vi "Winkel_ISO_bestimmen.vi"(8 "Fehler in":errorcluster, 11 "Cluster in":T1={"Initialisierung"={"Online?"=FALSE, "Grundpfad"=path "", "Kamera Oben"="", "IP-Adresse Flüssiglinse"="", "Flüssiglinse"=refnum, "Kamera Unten"="", "IP-Adresse SPS"="", "SPS-Verbindung"={"TCP Connection Ref"=refnum, "IP address"="", "timeout ms"=5000, "Connected?"=FALSE, "PLC Type"=enum."S7 1200", "Rack S7 400"=0, "Slot S7 400"=0, "PDU Size"=0, "connection semaphore"=refnum}, "IP-Adresse Lichtgitter"="", "Lichtgitter"=refnum, "Skalierungsfaktor"=0.0, "Bilder Oben"=[], "Bild Unten"=refnum, "Bild Ausschnitt Unten"=refnum}, "Einstellungen"={"Gesamtablauf gestartet"=FALSE, "i. O. Bilder speichern"=FALSE, "Bildspeicherung Offline"=FALSE, "Ausgewähltes Offline-Datum"="", "Ausgewähltes Offline-Teil"="", "Speicherpfad Bilder"=path ""}, "Artikeldaten"={"Artikelnummer"="", "Fertigungsauftrag"="", "Muster ISO"=refnum, "Belichtungszeit Referenzmarken"=0.0, "Fokus Referenzmarken"=0.0, "Belichtungszeit ISO"=0.0, "Fokus ISO"=0.0, "Belichtungszeit Unten"=0.0, "Kontaktanzahl"=0, "Aktueller Kontakt"=0, "Kontaktposition"={"x"=0.0, "y"=0.0}, "ISO-Muster nicht vorhanden"=FALSE, "Winkel ISO"=0.0, "Mittelpunkt ISO"={"x"=0.0, "y"=0.0}}, "Werte Kamera Oben"={"Koordinatensystem"={"Punkt x-Achse"={"X"=0.0, "Y"=0.0}, "Ursprung"={"X"=0.0, "Y"=0.0}, "Punkt y-Achse"={"X"=0.0, "Y"=0.0}}, "Position Kontakt"={"x"=0.0, "y"=0.0}, "Durchmesser Loch"=0.0, "Winkel Kontakt"=0.0, "Position Kontakt umgerechnet"={"x"=0.0, "y"=0.0}}, "Werte Kamera Unten"={"Prüfung Unten n. i. O."=FALSE}, "Werte Lichtgitter"={"Messwerte Referenzmarken"=[], "Mittelpunkt Referenzmarken"={"x"=0.0, "y"=0.0}, "Messwerte Kontakt"=[], "Offset"={"x"=0.0, "y"=0.0}}, "Rückmeldungen"={"Koordinaten ermittelt"=FALSE, "Vermessung Lichtgitter fertig"=FALSE, "Nachkontrolle Kamera Unten fertig"=FALSE}, "Fehler"={"Referenzen nicht gefunden"=FALSE, "Kontakt nicht gefunden"=FALSE, "Referenzen nicht in Lichtgitter"=FALSE, "Kontakt zu groß"=FALSE, "Kontakt zu klein"=FALSE}, "Statistik"={"Statistiken"=[]}, "Timer"={"Timer Start Position"=0, "Timer Start Lichtgitter"=0, "Timer Start Kamera Unten"=0}}) -> (0 "Fehler out":errorcluster, 2 "Polbild i.O.":bool, 3 "Cluster out":T1={"Initialisierung"={"Online?"=FALSE, "Grundpfad"=path "", "Kamera Oben"="", "IP-Adresse Flüssiglinse"="", "Flüssiglinse"=refnum, "Kamera Unten"="", "IP-Adresse SPS"="", "SPS-Verbindung"={"TCP Connection Ref"=refnum, "IP address"="", "timeout ms"=5000, "Connected?"=FALSE, "PLC Type"=enum."S7 1200", "Rack S7 400"=0, "Slot S7 400"=0, "PDU Size"=0, "connection semaphore"=refnum}, "IP-Adresse Lichtgitter"="", "Lichtgitter"=refnum, "Skalierungsfaktor"=0.0, "Bilder Oben"=[], "Bild Unten"=refnum, "Bild Ausschnitt Unten"=refnum}, "Einstellungen"={"Gesamtablauf gestartet"=FALSE, "i. O. Bilder speichern"=FALSE, "Bildspeicherung Offline"=FALSE, "Ausgewähltes Offline-Datum"="", "Ausgewähltes Offline-Teil"="", "Speicherpfad Bilder"=path ""}, "Artikeldaten"={"Artikelnummer"="", "Fertigungsauftrag"="", "Muster ISO"=refnum, "Belichtungszeit Referenzmarken"=0.0, "Fokus Referenzmarken"=0.0, "Belichtungszeit ISO"=0.0, "Fokus ISO"=0.0, "Belichtungszeit Unten"=0.0, "Kontaktanzahl"=0, "Aktueller Kontakt"=0, "Kontaktposition"={"x"=0.0, "y"=0.0}, "ISO-Muster nicht vorhanden"=FALSE, "Winkel ISO"=0.0, "Mittelpunkt ISO"={"x"=0.0, "y"=0.0}}, "Werte Kamera Oben"={"Koordinatensystem"={"Punkt x-Achse"={"X"=0.0, "Y"=0.0}, "Ursprung"={"X"=0.0, "Y"=0.0}, "Punkt y-Achse"={"X"=0.0, "Y"=0.0}}, "Position Kontakt"={"x"=0.0, "y"=0.0}, "Durchmesser Loch"=0.0, "Winkel Kontakt"=0.0, "Position Kontakt umgerechnet"={"x"=0.0, "y"=0.0}}, "Werte Kamera Unten"={"Prüfung Unten n. i. O."=FALSE}, "Werte Lichtgitter"={"Messwerte Referenzmarken"=[], "Mittelpunkt Referenzmarken"={"x"=0.0, "y"=0.0}, "Messwerte Kontakt"=[], "Offset"={"x"=0.0, "y"=0.0}}, "Rückmeldungen"={"Koordinaten ermittelt"=FALSE, "Vermessung Lichtgitter fertig"=FALSE, "Nachkontrolle Kamera Unten fertig"=FALSE}, "Fehler"={"Referenzen nicht gefunden"=FALSE, "Kontakt nicht gefunden"=FALSE, "Referenzen nicht in Lichtgitter"=FALSE, "Kontakt zu groß"=FALSE, "Kontakt zu klein"=FALSE}, "Statistik"={"Statistiken"=[]}, "Timer"={"Timer Start Position"=0, "Timer Start Lichtgitter"=0, "Timer Start Kamera Unten"=0}})   [LabVIEW 2024]
uses:
  Typdefinitionen/Cluster.ctl
  <vilib>/userDefined/High Color/IMAQdx.ctl
  <vilib>/DATA AHEAD/SP7/typedefs/S7 Connection.ctl
  <vilib>/DATA AHEAD/SP7/typedefs/PLC Type.ctl
  <vilib>/vision/Image Controls.llb/IMAQ Image.ctl
  Typdefinitionen/Koordinatensystem.ctl
  Typdefinitionen/Statistik.ctl
  <vilib>/vision/NI_Vision_Development_Module.lvlib
  <vilib>/DATA AHEAD/SP7/SP7.lvlib
panel:
  out "Number of Matches":i32
  out "Zeit Pattern Matching":u32
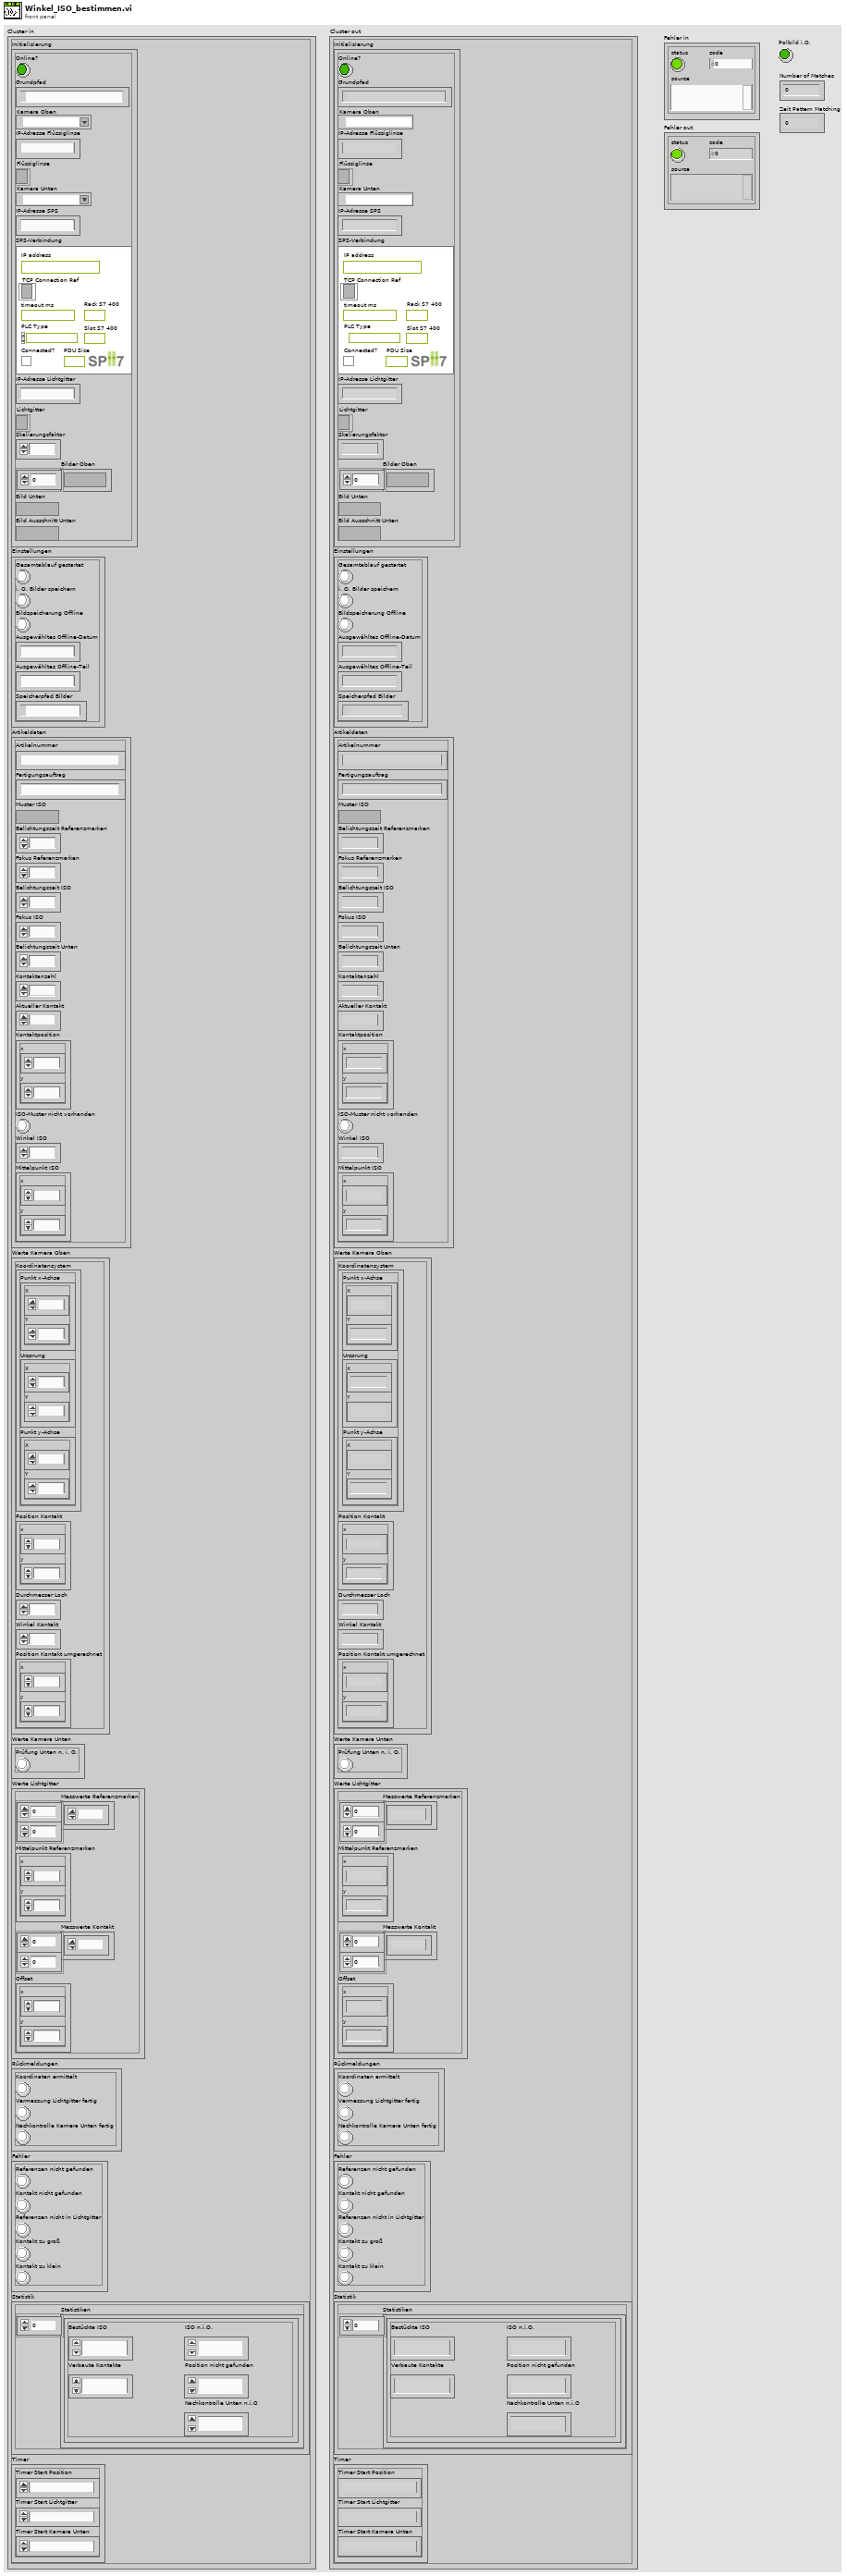
[diagram p1: front panel]
types:
  T1 = typedef "Cluster.ctl" = cluster{"Initialisierung":cluster{"Online?":bool, "Grundpfad":path, "Kamera Oben":T2, "IP-Adresse Flüssiglinse":string, "Flüssiglinse":refnum<k5>, "Kamera Unten":T2, "IP-Adresse SPS":string, "SPS-Verbindung":T3, "IP-Adresse Lichtgitter":string, "Lichtgitter":refnum<k5>, "Skalierungsfaktor":dbl, "Bilder Oben":T6[], "Bild Unten":T6, "Bild Ausschnitt Unten":T6}, "Einstellungen":cluster{"Gesamtablauf gestartet":bool, "i. O. Bilder speichern":bool, "Bildspeicherung Offline":bool, "Ausgewähltes Offline-Datum":string, "Ausgewähltes Offline-Teil":string, "Speicherpfad Bilder":path}, "Artikeldaten":cluster{"Artikelnummer":string, "Fertigungsauftrag":string, "Muster ISO":T6, "Belichtungszeit Referenzmarken":dbl, "Fokus Referenzmarken":dbl, "Belichtungszeit ISO":dbl, "Fokus ISO":dbl, "Belichtungszeit Unten":dbl, "Kontaktanzahl":u32, "Aktueller Kontakt":i16, "Kontaktposition":cluster{"x":sgl, "y":sgl}, "ISO-Muster nicht vorhanden":bool, "Winkel ISO":sgl, "Mittelpunkt ISO":cluster{"x":dbl, "y":dbl}}, "Werte Kamera Oben":cluster{"Koordinatensystem":T7, "Position Kontakt":cluster{"x":dbl, "y":dbl}, "Durchmesser Loch":dbl, "Winkel Kontakt":dbl, "Position Kontakt umgerechnet":cluster{"x":dbl, "y":dbl}}, "Werte Kamera Unten":cluster{"Prüfung Unten n. i. O.":bool}, "Werte Lichtgitter":cluster{"Messwerte Referenzmarken":dbl[][], "Mittelpunkt Referenzmarken":cluster{"x":dbl, "y":dbl}, "Messwerte Kontakt":dbl[][], "Offset":cluster{"x":dbl, "y":dbl}}, "Rückmeldungen":cluster{"Koordinaten ermittelt":bool, "Vermessung Lichtgitter fertig":bool, "Nachkontrolle Kamera Unten fertig":bool}, "Fehler":cluster{"Referenzen nicht gefunden":bool, "Kontakt nicht gefunden":bool, "Referenzen nicht in Lichtgitter":bool, "Kontakt zu groß":bool, "Kontakt zu klein":bool}, "Statistik":cluster{"Statistiken":T8[]}, "Timer":cluster{"Timer Start Position":u32, "Timer Start Lichtgitter":u32, "Timer Start Kamera Unten":u32}}
  T2 = typedef "IMAQdx.ctl" = refnum<k21>
  T3 = typedef "SP7.lvlib/S7 Connection.ctl" = cluster{"TCP Connection Ref":refnum<k5>, "IP address":string, "timeout ms":i32, "Connected?":bool, "PLC Type":T4, "Rack S7 400":u8, "Slot S7 400":u8, "PDU Size":u16, "connection semaphore":T5}
  T4 = typedef "SP7.lvlib/PLC Type.ctl" = enum16{"S7 200", "S7 300/400", "S7 1200", "S7 1500", "LOGO!8"}
  T5 = typedef "Semaphore RefNum" = refnum<k1>
  T6 = typedef "IMAQ Image.ctl" = refnum<image>
  T7 = typedef "Koordinatensystem.ctl" = cluster{"Punkt x-Achse":cluster{"X":sgl, "Y":sgl}, "Ursprung":cluster{"X":sgl, "Y":sgl}, "Punkt y-Achse":cluster{"X":sgl, "Y":sgl}}
  T8 = typedef "Statistik.ctl" = cluster{"Bestückte ISO":u32, "Verbaute Kontakte":u32, "ISO n.i.O.":u32, "Nachkontrolle Unten n.i.O":u32, "Position nicht gefunden":u32}
  T9 = cluster{"Number of Matches Requested":i32, "Minimum Match Score":sgl, "Angle Ranges":cluster{"Start Angle":sgl, "End Angle":sgl}[]}
  T10 = cluster{"Position":cluster{"x":sgl, "y":sgl}, "Angle":sgl, "Scale":sgl, "Score":sgl, "Bounding Box":cluster{"x":sgl, "y":sgl}[]}[]
  T11 = cluster{"Position":cluster{"x":sgl, "y":sgl}, "Angle":sgl, "Scale":sgl, "Score":sgl, "Bounding Box":cluster{"x":sgl, "y":sgl}[]}
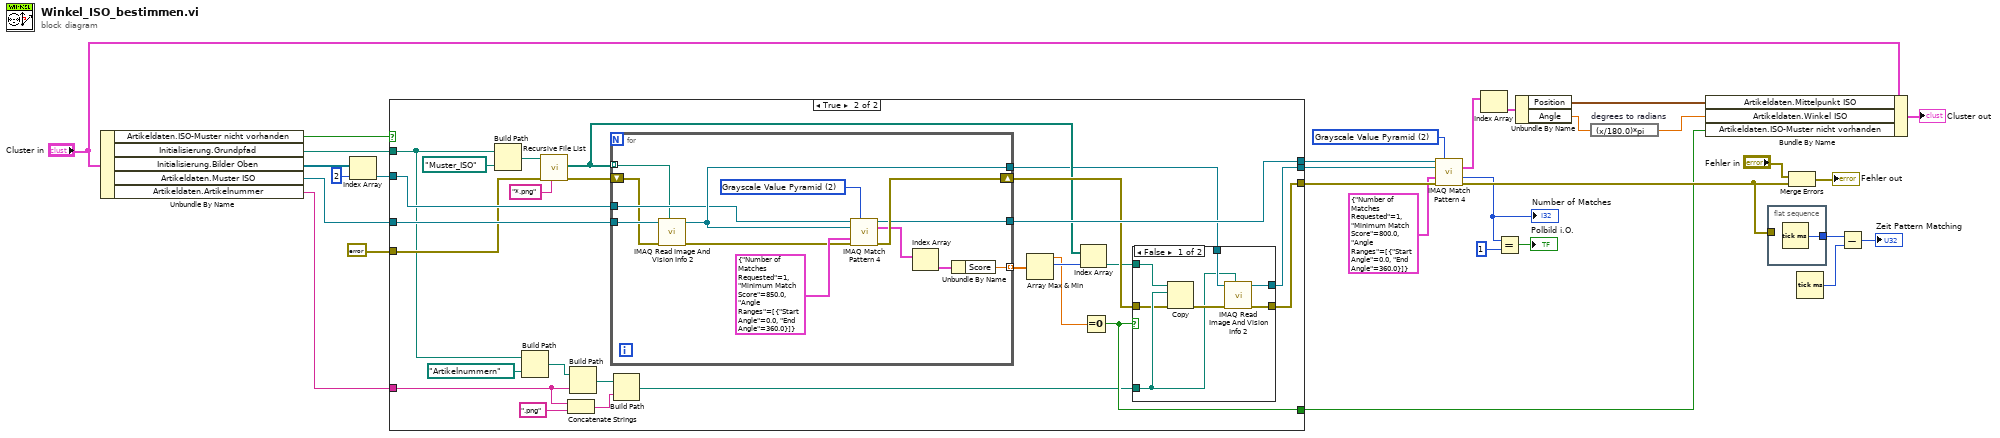
[diagram p0: block diagram]
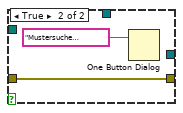
[diagram p3: hidden frame]
diagram:
  w4 = 2 items=["All", "Low Discrepancy Sampling", "Grayscale Value Pyramid", "Gradients Pyramid"] ("Algorithm")
  n1 = Unbundle By Name("Cluster in") -> ("Artikeldaten.ISO-Muster nicht vorhanden"=w19:bool, "Initialisierung.Grundpfad"=w18:path, "Initialisierung.Bilder Oben"=w17:T6[], "Artikeldaten.Muster ISO"=w15:T6, "Artikeldaten.Artikelnummer"=w13:string)
  n2 = Index Array(array=w17, index=2) -> (element=w16:T6)
  n3 = case shown="True" w19 {
    tunnel: w18 -> [_ w51]
    tunnel: [w31 w44] -> w6
    tunnel: w15 -> [w32 w56]
    tunnel: [w32 w39] -> w7
    tunnel: w16 -> [w33 w55]
    tunnel: errorcluster {"status"=FALSE, "code"=0, "source"=""} ("error in") -> [w31 w53]
    tunnel: [w33 w52] -> w14
    tunnel: w13 -> [_ w37]
    tunnel: [_ w41] -> w10
    frame False {
    }
    frame True {
      n4 = Build Path(base path=w51, name or relative path=path "Muster_ISO") -> (appended path=w58:path)
      n5 = Build Path(base path=w51, name or relative path=path "Artikelnummern") -> (appended path=w49:path)
      n6 = call <vilib>:"Recursive File List.vi"("pattern"="*.png", "error in (no error)"=w53, "Folder Path"=w58) -> ("error out"=w54:errorcluster, "All Files in Dir"=w45:path[])  [unwired: 4 in, 3 out]
      n7 = Concatenate Strings(w37, ".png" ("string")) -> (w35:string)
      n8 = Build Path(base path=w49, name or relative path=w37) -> (appended path=w36:path)
      n9 = for {
        tunnel: w45 -> [w63] mode=indexing
        tunnel: w56 -> [w70]
        tunnel: [w69] -> w40
        tunnel: w55 -> [w68]
        shift-right: [w65] -> w48
        shift-left: w54 -> [w67]
        tunnel: [w64] -> w52
        tunnel: [w60] -> w47 mode=indexing
        w71 = 2 items=["All", "Low Discrepancy Sampling", "Grayscale Value Pyramid", "Gradients Pyramid"] ("Algorithm")
        n10 = call "IMAQ Read Image And Vision Info 2"("File Path"=w63, "error in (no error)"=w67, "Image"=w70) -> ("error out"=w66:errorcluster, "Image Out"=w69:T6)  [unwired: 6 in, 1 out]
        n11 = call "IMAQ Match Pattern 4"("Image"=w68, "Algorithm"=w71, "Template Image"=w69, "Parameters"=T9 {"Number of Matches Requested"=1, "Minimum Match Score"=850.0, "Angle Ranges"=[{"Start Angle"=0.0, "End Angle"=360.0}]}, "error in (no error)"=w66) -> ("Image (duplicate)"=w64:T6, "Matches (pixel)"=w62:T10, "error out"=w65:errorcluster)  [unwired: 6 in, 2 out]
        n12 = Index Array(array=w62) -> (element=w61:T11)  [unwired: 1 in]
        n13 = Unbundle By Name(w61) -> ("Score"=w60:sgl)
      }
      n14 = Build Path(base path=w36, name or relative path=w35) -> (appended path=w34:path)
      n15 = Array Max & Min(array=w47) -> (max value=w42:sgl, max index (indices)=w46:i32)  [unwired: 2 out]
      n16 = Index Array(array=w45, index=w46) -> (element=w43:path)
      n17 = Equal To 0?(x=w42) -> (x = 0?=w41:bool)
      n18 = case shown="False" w41 {
        tunnel: w48 -> [w73 w81]
        tunnel: [w77 w81] -> w44
        tunnel: w43 -> [w79 _]
        tunnel: w40 -> [w76 _]
        tunnel: [w75 _] -> w39
        tunnel: w34 -> [w74 _]
        frame False {
          n19 = Copy(8:w73, 10:w74, 11:w79) -> (0:w78:errorcluster)  [unwired: 2 in, 2 out]
          n20 = call "IMAQ Read Image And Vision Info 2"("File Path"=w74, "error in (no error)"=w78, "Image"=w76) -> ("error out"=w77:errorcluster, "Image Out"=w75:T6)  [unwired: 6 in, 1 out]
        }
        frame True {
          n21 = One Button Dialog(message="Mustersuche fehlgeschlagen!") -> ()  [unwired: 1 in, 1 out]
        }
      }
    }
  }
  n22 = call "IMAQ Match Pattern 4"("Image"=w14, "Algorithm"=w4, "Template Image"=w7, "Parameters"=T9 {"Number of Matches Requested"=1, "Minimum Match Score"=800.0, "Angle Ranges"=[{"Start Angle"=0.0, "End Angle"=360.0}]}, "error in (no error)"=w6) -> ("Matches (pixel)"=w24:T10, "Number of Matches"=w3:i32, "error out"=w12:errorcluster)  [unwired: 6 in, 2 out]
  "Number of Matches" <- w3
  n23 = Index Array(array=w24) -> (element=w23:T11)  [unwired: 1 in]
  n24 = Equal?(x=w3, y=1) -> (x = y?=→"Polbild i.O.":bool)
  n25 = Unbundle By Name(w23) -> ("Position"=w2:cluster{"x":sgl, "y":sgl}, "Angle"=w26:sgl)
  n26 = expression code="(x/180.0)*pi" "degrees to radians"(w26) -> (w1:sgl)
  n27 = Bundle By Name(cluster="Cluster in", "Artikeldaten.Mittelpunkt ISO"=w2, "Artikeldaten.Winkel ISO"=w1, "Artikeldaten.ISO-Muster nicht vorhanden"=w10) -> (→"Cluster out":T1)
  n28 = flat-sequence {
    tunnel: [w82] -> w22
    tunnel: w12 -> [_]
    frame #0 {
      n29 = Tick Count (ms)() -> (millisecond timer value=w82:u32)
    }
  }
  n30 = Merge Errors("Fehler in", w12) -> (→"Fehler out":errorcluster)
  n31 = Tick Count (ms)() -> (millisecond timer value=w21:u32)
  n32 = Subtract(x=w22, y=w21) -> (x-y=→"Zeit Pattern Matching":u32)
